vi "BarrelTrackerTeam.vi"() -> ()   [LabVIEW 2012]
uses:
  <vilib>/vision/Image Controls.llb/IMAQ Image.ctl
panel:
  in  "Image In":T1=refnum
  in  "stop":bool
  in  "Template File Path (Pattern Matching)":path=path "C:/Users/solorzaa/Desktop/Barrels/Templates/barrelTemp3.png"
  out "Input Image":T1(plugin-control)
  out "Processed Image":T1(plugin-control)
  in  "Loop Delay (ms)":u32(slide)=200 scale=0.0..250.0
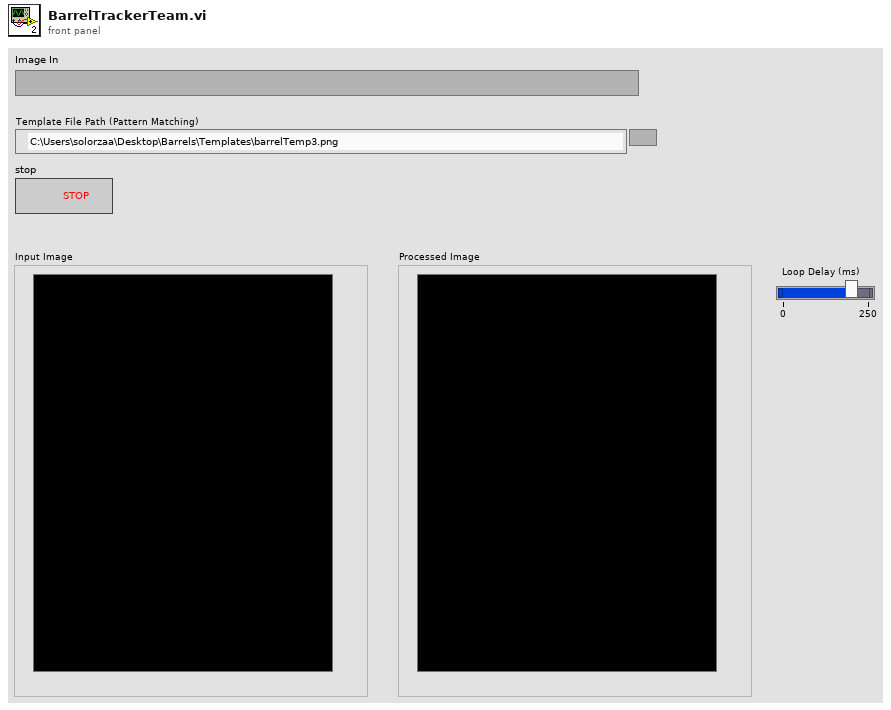
[diagram p1: front panel]
types:
  T1 = typedef "IMAQ Image.ctl" = refnum<image>
  T2 = cluster{"Position":cluster{"x":sgl, "y":sgl}, "Angle":sgl, "Scale":sgl, "Score":sgl, "Bounding Box":cluster{"x":sgl, "y":sgl}[]}[]
  T3 = typedef "ROI Descriptor" = cluster{"Global Rectangle":i32[], "Contours":cluster{"ID":enum32{"External", "Internal"}, "Type":u32, "Coordinates":i32[]}[]}
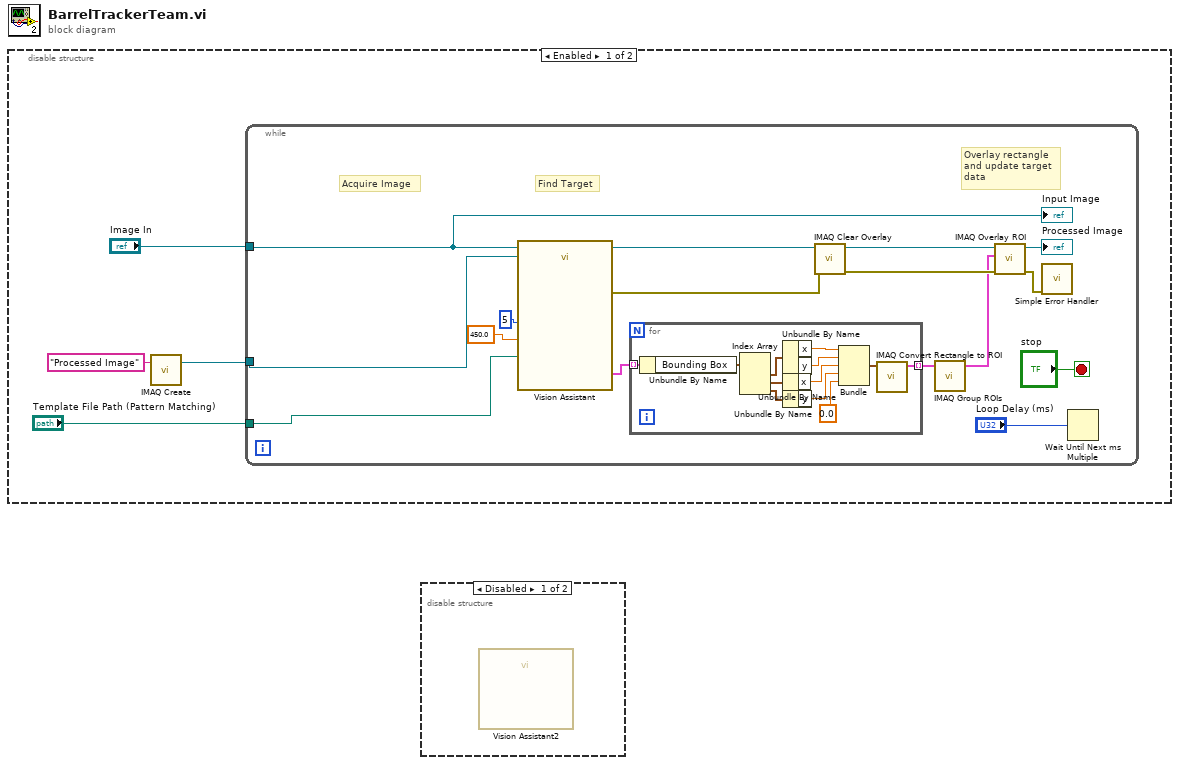
[diagram p0: block diagram]
diagram:
  n1 = disable-structure shown="Enabled" {
    frame Enabled {
      n2 = call "IMAQ Create"("Image Name"="Processed Image") -> ("New Image"=w3:T1)  [unwired: 3 in, 2 out]
      n3 = while {
        tunnel: w3 -> [w20]
        tunnel: "Image In" -> [w7]
        tunnel: "Template File Path (Pattern Matching)" -> [w6]
        stop <- "stop" stop-if-true
        # "Overlay rectangle\nand update target\ndata"
        # "Find Target"
        # "Acquire Image"
        n4 = call "Vision Assistant"("Image In"=w7, "Image Dst"=w20, "Number of Matches Requested (Pattern Matching)"=5 ("Number of Matches Requested (Pattern Matching 1)"), "Minimum Match Score (Pattern Matching)"=sgl 450.0 ("Minimum Match Score"), "Template File Path (Pattern Matching)"=w6) -> ("Image Out"=w19:T1, "Matches (Pattern Matching)"=w11:T2, "error out"=w17:errorcluster)  [unwired: 1 in, 19 out]
        n5 = for {
          tunnel: w11 -> [w32] mode=indexing
          tunnel: [w23] -> w10 mode=indexing
          n6 = Unbundle By Name(w32) -> ("Bounding Box"=w31:cluster{"x":sgl, "y":sgl}[])
          n7 = Index Array(array=w31) -> (element #1=w30:cluster{"x":sgl, "y":sgl}, element #2=w29:cluster{"x":sgl, "y":sgl}, element #3=w22:cluster{"x":sgl, "y":sgl})  [unwired: 3 in]
          n8 = Unbundle By Name(w30) -> ("x"=w28:sgl, "y"=w27:sgl)
          n9 = Unbundle By Name(w29) -> ("x"=w26:sgl)
          n10 = Unbundle By Name(w22) -> ("y"=w21:sgl)
          n11 = Bundle("x"=w28, "y"=w27, "x"=w26, "y"=w21, 0.0) -> (w24:cluster{"x":sgl, "y":sgl, "x":sgl, "y":sgl, dbl})  [unwired: 1 out]
          n12 = call "IMAQ Convert Rectangle to ROI"("Rectangle"=w24) -> ("ROI Descriptor"=w23:T3)  [unwired: 1 in, 8 out]
        }
        n13 = call "IMAQ Clear Overlay"("error in (no error)"=w17, "Image"=w19) -> ("error out"=w16:errorcluster, "Image Out"=w8:T1)  [unwired: 1 in, 7 out]
        n14 = call "IMAQ Group ROIs"("ROI Descriptors"=w10) -> ("ROI Descriptor out"=w9:T3)  [unwired: 1 in, 3 out]
        n15 = call "IMAQ Overlay ROI"("error in (no error)"=w16, "ROI Descriptor"=w9, "Image"=w8) -> ("error out"=w14:errorcluster, "Image Out"=→"Processed Image":T1)  [unwired: 3 in, 4 out]
        n16 = call <vilib>:"Simple Error Handler.vi"("error in (no error)"=w14) -> ()  [unwired: 1 in, 8 out]
        n17 = Wait Until Next ms Multiple(millisecond multiple="Loop Delay (ms)") -> ()  [unwired: 1 out]
        "Input Image" <- w7
      }
    }
    frame Disabled {
    }
  }
  n18 = disable-structure shown="Disabled" {
    frame Disabled {
      n19 = call "Vision Assistant2"() -> ()  [unwired: 26 in, 2 out]
    }
    frame Disabled {
    }
  }
